vi "Previous_Data_log.vi"(7 "?":enum16{"Write", "Read"}(ring), 8 "error in (no error)":errorcluster, 10 "Data IN":string[](array[string]), 11 "file path (dialog if empty)":path=path "E:/Work/NI Vision/Tata_ficoso Data Logging Software/XBA/XBA ORVM V2/Data/Previous_Part_data.csv") -> (0 "error out":errorcluster, 3 "all rows":string[][](array[string]))   [LabVIEW 2017]
uses:
  <vilib>/Utility/file.llb/Read Delimited Spreadsheet (string).vi
  <vilib>/Utility/file.llb/Write Delimited Spreadsheet (string).vi
panel:
  out "subarray":string[](array[string])
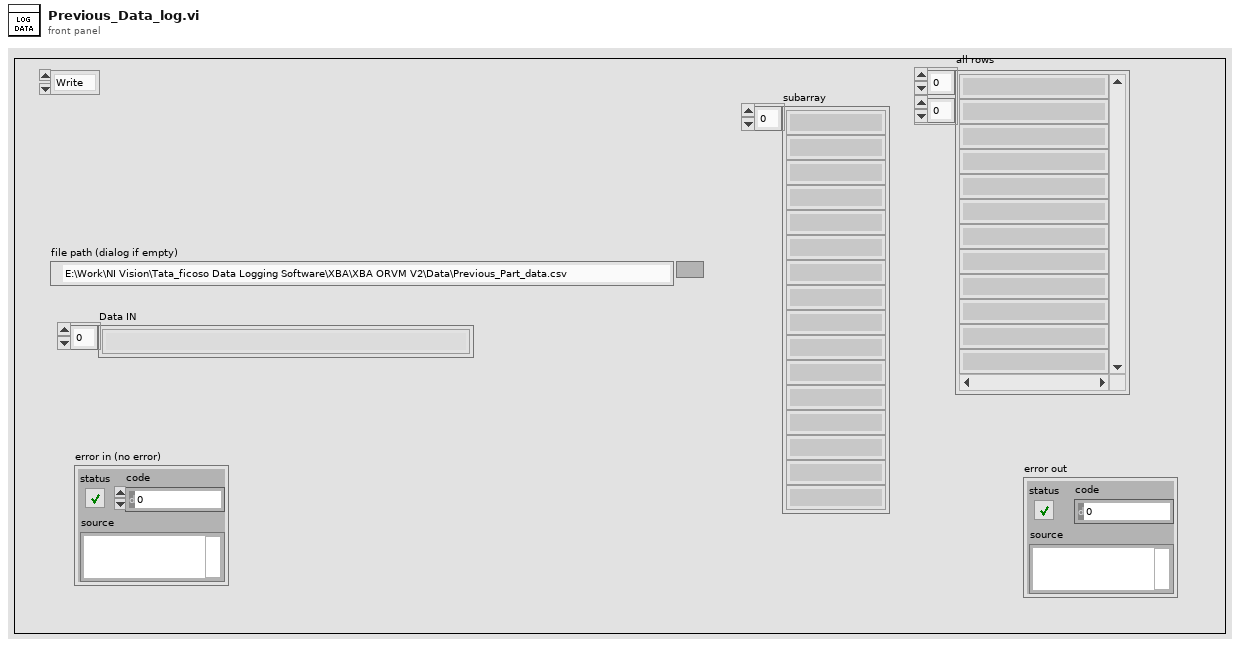
[diagram p1: front panel]
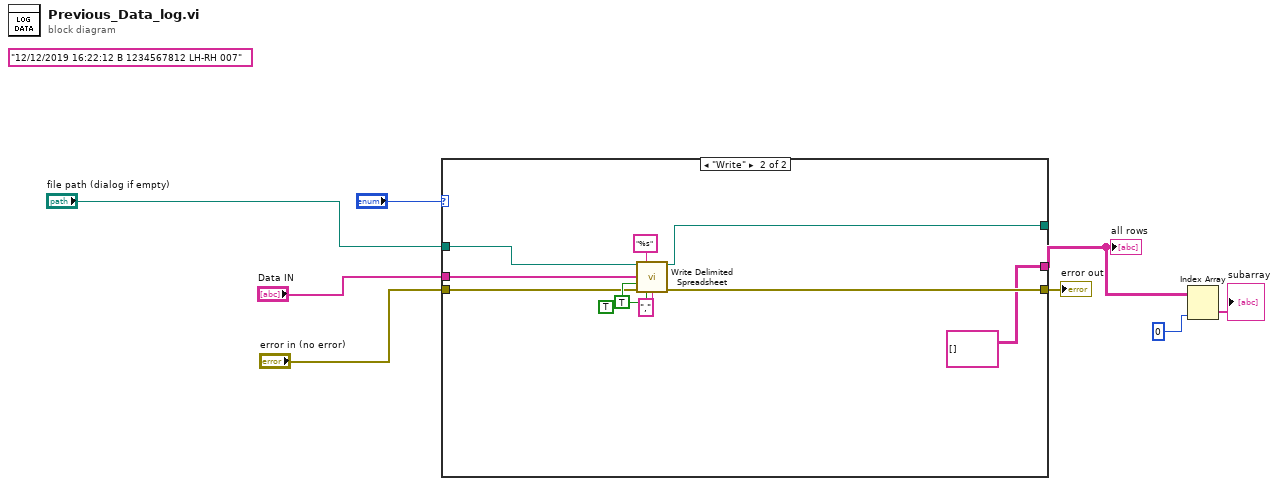
[diagram p0: block diagram]
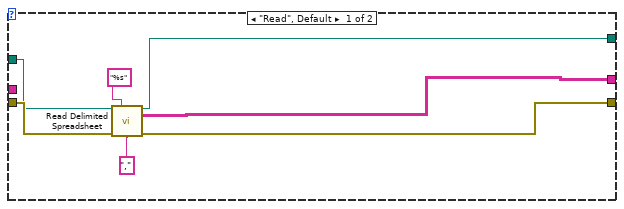
[diagram p2: hidden frame]
diagram:
  (unwired) "12/12/2019 16:22:12 B 1234567812 LH-RH 007" ("string")
  n1 = case shown="\"Write\"" "?" {
    tunnel: "Data IN" -> [_ w22]
    tunnel: "error in (no error)" -> [w13 w21]
    tunnel: [w11 w20] -> w6
    tunnel: "file path (dialog if empty)" -> [w12 w19]
    tunnel: [w10 w18] -> _
    tunnel: [w9 string[][] [] ("all rows")] -> w2
    frame "Read", Default {
      n2 = call-poly <vilib>:"Read Delimited Spreadsheet.vi"("file path (dialog if empty)"=w12, "format (%s)"="%s", "error in (no error)"=w13, "delimiter (\\t)"="," ("delimiter (\\t)")) -> ("new file path (Not A Path if cancelled)"=w10:path, "all rows"=w9:string[][], "error out"=w11:errorcluster)  [unwired: 6 in, 3 out]
    }
    frame "Write" {
      n3 = call-poly <vilib>:"Write Delimited Spreadsheet.vi"("file path (dialog if empty)"=w19, "format (%s)"="%s", "1D data"=w22, "append to file? (new file:F)"=TRUE, "error in (no error)"=w21, "transpose? (no:F)"=TRUE, "delimiter (\\t)"="," ("delimiter (\\t)")) -> ("new file path (Not A Path if cancelled)"=w18:path, "error out"=w20:errorcluster)  [unwired: 7 in]
    }
  }
  "all rows" <- w2
  "error out" <- w6
  n4 = Index Array(array=w2, index (col)=0 ("disabled index (col)")) -> (element=→"subarray":string[])  [unwired: 1 in]
